vi "工單號碼Table Add.vi"(11 "Work No":refnum<vi>) -> ()   [LabVIEW 2019]
uses:
  Ctrl/Table Save.ctl
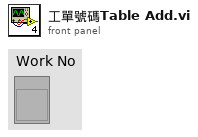
[diagram p1: front panel]
types:
  T1 = typedef "Table Save.ctl" = enum16{"initial", "Add", "Write", "Replace", "Delete", "REad", "RedTable", "Load"}
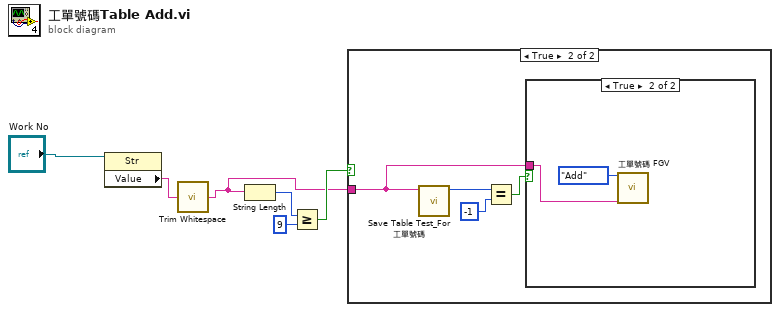
[diagram p0: block diagram]
diagram:
  n1 = property class="Str"(reference="Work No") -> ("Value"=w3:string)  [unwired: 1 in, 2 out]
  n2 = call <vilib>:"Trim Whitespace.vi"("string"=w3) -> ("trimmed string"=w2:string)  [unwired: 1 in]
  n3 = String Length(string=w2) -> (length=w6:i32)
  n4 = Greater Or Equal?(x=w6, y=9) -> (x >= y?=w4:bool)
  n5 = case shown="True" w4 {
    tunnel: w2 -> [_ w8]
    frame False {
    }
    frame True {
      n6 = call "Save Table Test_For 工單號碼.vi"("工單號碼"=w8) -> ("條碼的Index"=w9:i32)  [unwired: 9 in, 1 out]
      n7 = Equal?(x=w9, y=-1) -> (x = y?=w7:bool)
      n8 = case shown="True" w7 {
        tunnel: w8 -> [_ w11]
        frame False {
        }
        frame True {
          n9 = call "工單號碼 FGV.vi"("Action"=Table_Save."Add", "工單號碼"=w11) -> ()  [unwired: 10 in, 8 out]
        }
      }
    }
  }
